vi "ConfigureSyringeBD.vi"(0 "object in":refnum<class "CetoniPump.lvclass">, 2 "Syringe":T1(ring), 5 "error in (no error)":errorcluster) -> (14 "object out":refnum<class "CetoniPump.lvclass">, 19 "error out":errorcluster)   [LabVIEW 2021, in "CetoniPump.lvclass"]
uses:
  CetoniPump.lvclass
  CetoniPump.lvclass/CetoniPump.ctl
panel:
  out "x*y":dbl
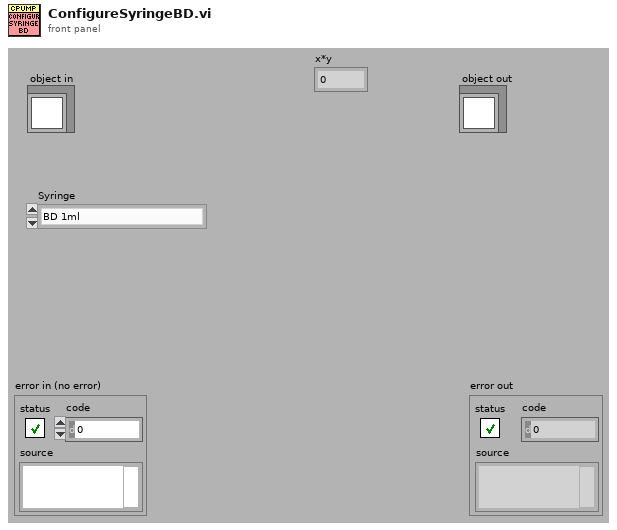
[diagram p1: front panel]
types:
  T1 = enum16{"BD 1ml", "BD 3ml", "BD 5ml", "BD 10ml", "BD 20ml", "BD 30ml", "BD 50ml", "HSW 1ml"}
  T2 = cluster{"Maximum Piston Stroke (mm)":dbl, "Inner Diameter (mm)":dbl}
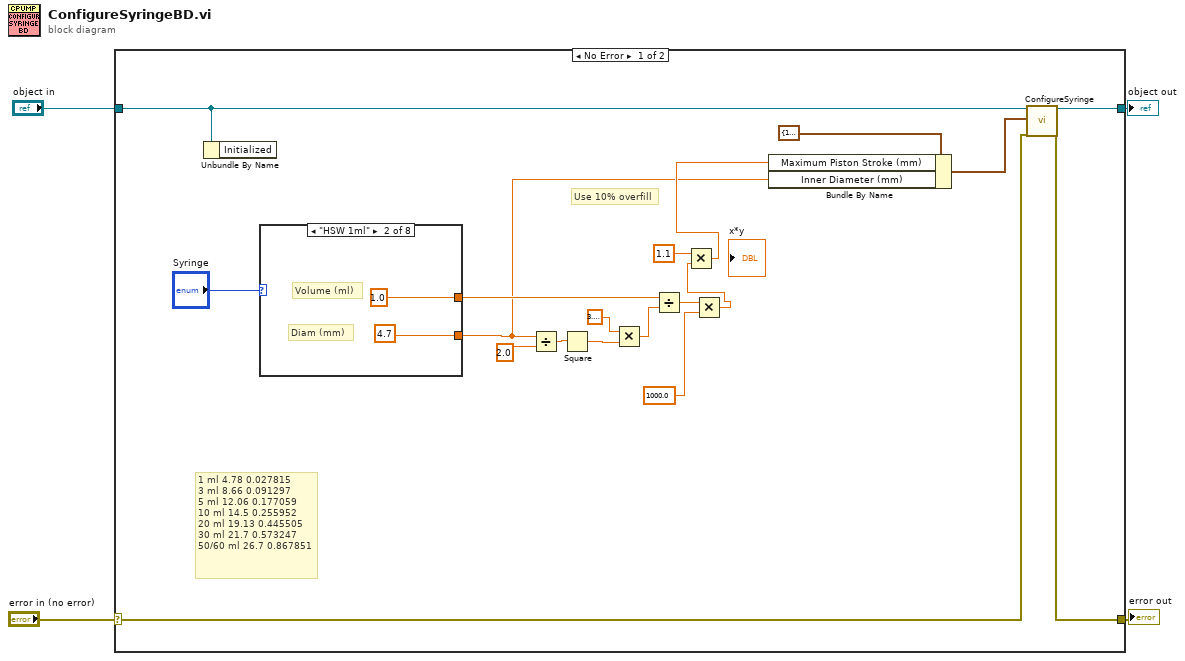
[diagram p0: block diagram]
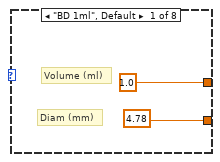
[diagram p2: hidden frame]
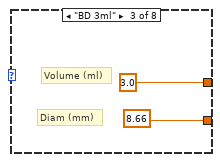
[diagram p3: hidden frame]
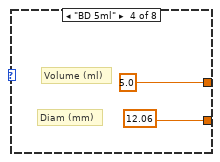
[diagram p4: hidden frame]
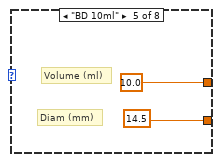
[diagram p5: hidden frame]
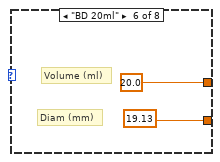
[diagram p6: hidden frame]
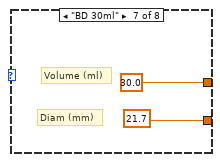
[diagram p7: hidden frame]
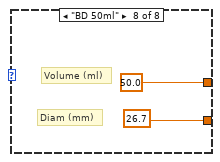
[diagram p8: hidden frame]
diagram:
  n1 = case shown="No Error" "error in (no error)" {
    selector: "error in (no error)" -> [w6 w41]
    tunnel: [w5 w41] -> w3
    tunnel: [w11 w40] -> w1
    tunnel: "object in" -> [w23 w40]
    frame No Error {
      # "Use 10% overfill"
      # "1 ml 4.78 0.027815\n3 ml 8.66 0.091297\n5 ml 12.06 0.177059\n10 ml 14.5 0.255952\n20 ml 19.13 0.445505\n30 ml 21.7 0.573247\n50/60 ml 26.7 0.867851"
      n2 = Unbundle By Name(w23) -> ()  [unwired: 1 out]
      n3 = case shown="\"HSW 1ml\"" "Syringe" {
        tunnel: [1.0 1.0 3.0 5.0 10.0 20.0 30.0 50.0] -> w15
        tunnel: [4.78 4.7 8.66 12.06 14.5 19.13 21.7 26.7] -> w8
        frame "BD 1ml", Default {
          # "Diam (mm)"
          # "Volume (ml)"
        }
        frame "HSW 1ml" {
          # "Diam (mm)"
          # "Volume (ml)"
        }
        frame "BD 3ml" {
          # "Diam (mm)"
          # "Volume (ml)"
        }
        frame "BD 5ml" {
          # "Diam (mm)"
          # "Volume (ml)"
        }
        frame "BD 10ml" {
          # "Diam (mm)"
          # "Volume (ml)"
        }
        frame "BD 20ml" {
          # "Diam (mm)"
          # "Volume (ml)"
        }
        frame "BD 30ml" {
          # "Diam (mm)"
          # "Volume (ml)"
        }
        frame "BD 50ml" {
          # "Diam (mm)"
          # "Volume (ml)"
        }
      }
      n4 = Divide(x=w8, y=2.0) -> (x/y=w20:dbl)
      n5 = Square(x=w20) -> (x^2=w19:dbl)
      n6 = Multiply(x=3.141592653589793, y=w19) -> (x*y=w16:dbl)
      n7 = Divide(x=w15, y=w16) -> (x/y=w13:dbl)
      n8 = Multiply(x=w13, y=1000.0) -> (x*y=w12:dbl)
      n9 = Multiply(x=1.1, y=w12) -> (x*y=w9:dbl)
      n10 = Bundle By Name(cluster=T2 {"Maximum Piston Stroke (mm)"=100.0, "Inner Diameter (mm)"=12.0} ("SyringeSettings"), "Maximum Piston Stroke (mm)"=w9, "Inner Diameter (mm)"=w8) -> (w7:T2)
      n11 = call-dynamic "ConfigureSyringe.vi"("object in"=w23, "SyringeSettings"=w7, "error in (no error)"=w6) -> ("object out"=w11:refnum<class "CetoniPump.lvclass">, "error out"=w5:errorcluster)  [unwired: 15 in]
    }
    frame Error {
    }
  }
  "error out" <- w3
  "object out" <- w1
